vi "LEDStateControl.vi"   [LabVIEW 2018]
uses:
  RobotStates.vi
  Inputs_DriverStation.vi
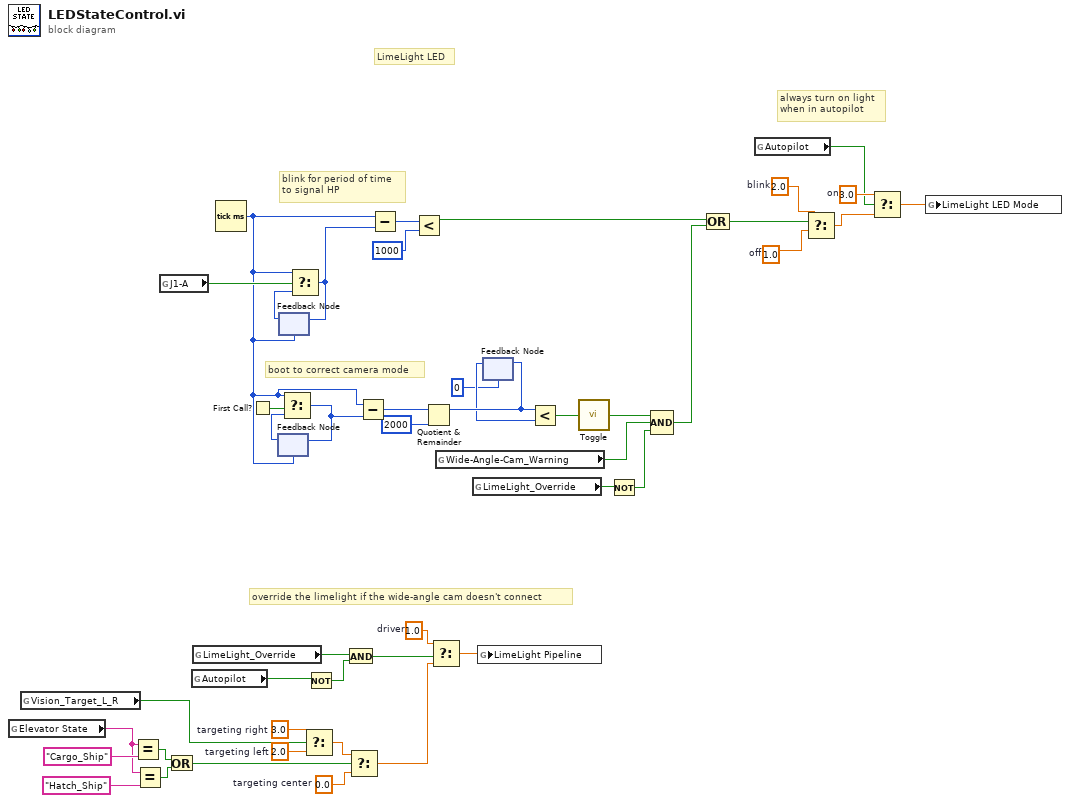
[diagram p0: block diagram]
diagram:
  w2 = 3.0  # targeting right
  w3 = 2.0  # targeting left
  w6 = 0.0  # targeting center
  w22 = 1.0  # driver
  w43 = 2.0  # blink
  w34 = 1.0  # off
  w45 = 3.0  # on
  # "override the limelight if the wide-angle cam doesn't connect"
  # "boot to correct camera mode"
  # "LimeLight LED"
  # "always turn on light\nwhen in autopilot"
  # "blink for period of time\nto signal HP"
  n1 = global read "RobotStates.vi" "Elevator State"() -> (w11:string)
  n2 = global read "Inputs_DriverStation.vi" "Vision_Target_L_R"() -> (w4:bool)
  n3 = Equal?(x=w11, y="Cargo_Ship") -> (x = y?=w8:bool)
  n4 = Equal?(x=w11, y="Hatch_Ship") -> (x = y?=w9:bool)
  n5 = global read "Inputs_DriverStation.vi" "J1-A"() -> (w42:bool)
  n6 = Or(x=w8, y=w9) -> (x .or. y?=w5:bool)
  n7 = global read "RobotStates.vi" "Autopilot"() -> (w14:bool)
  n8 = global read "Inputs_DriverStation.vi" "LimeLight_Override"() -> (w16:bool)
  n9 = Tick Count (ms)() -> (millisecond timer value=w30:u32)
  n10 = First Call?() -> (First Call?: T/F=w37:bool)
  n11 = feedback #1(w30) -> (w36:u32)
  n12 = feedback #2(w30) -> (w41:u32)
  n13 = Select(t=w30, s=w37, f=w36) -> (s? t:f=w31:u32)
  n14 = feedback-in #1(w31) -> ()
  n15 = Select(t=w30, s=w42, f=w41) -> (s? t:f=w40:u32)
  n16 = feedback-in #2(w40) -> ()
  n17 = Select(t=w2, s=w4, f=w3) -> (s? t:f=w7:dbl)
  n18 = Not(x=w14) -> (.not. x?=w13:bool)
  n19 = And(x=w16, y=w13) -> (x .and. y?=w15:bool)
  n20 = Select(t=w7, s=w5, f=w6) -> (s? t:f=w1:dbl)
  n21 = Subtract(x=w30, y=w31) -> (x-y=w25:u32)
  n22 = Subtract(x=w30, y=w40) -> (x-y=w39:u32)
  n23 = Less?(x=w39, y=u32 1000) -> (x < y?=w33:bool)
  n24 = Quotient & Remainder(x=w25, y=u32 2000) -> (x-y*floor(x/y)=w28:u32)  [unwired: 1 out]
  n25 = Select(t=w22, s=w15, f=w1) -> (s? t:f=w23:dbl)
  n26 = global read "Inputs_DriverStation.vi" "Wide-Angle-Cam_Warning"() -> (w19:bool)
  n27 = global read "Inputs_DriverStation.vi" "LimeLight_Override"() -> (w18:bool)
  n28 = global write "RobotStates.vi" "LimeLight Pipeline"(w23) -> ()
  n29 = feedback #3(u32 0) -> (w27:u32)
  n30 = feedback-in #3(w28) -> ()
  n31 = Less?(x=w28, y=w27) -> (x < y?=w24:bool)
  n32 = call "Toggle.vi"("Trigger"=w24) -> ("New Mode"=w21:bool)
  n33 = Not(x=w18) -> (.not. x?=w17:bool)
  n34 = Compound Arithmetic op=AND(w21, w19, w17) -> (w20:bool)
  n35 = Compound Arithmetic op=OR(w33, w20) -> (w32:bool)
  n36 = global read "RobotStates.vi" "Autopilot"() -> (w35:bool)
  n37 = Select(t=w43, s=w32, f=w34) -> (s? t:f=w44:dbl)
  n38 = Select(t=w45, s=w35, f=w44) -> (s? t:f=w46:dbl)
  n39 = global write "RobotStates.vi" "LimeLight LED Mode"(w46) -> ()
